vi "SCGlobVars.vi"() -> ()   [LabVIEW 2014]
uses:
  Controls/SPstate.ctl
panel:
  in  "SCerrorCount":u8
  in  "SCstate":T1
  in  "dwellTime":u32=2000000
  in  "stop":bool
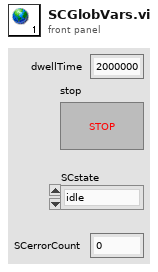
[diagram p1: front panel]
types:
  T1 = typedef "SPstate.ctl" = enum16{"idle", "scanning", "done", "error"}
diagram:
